vi "BuildPopupHelper.vi"(1 "new":T1(array[cluster]), 2 "main":T1(array[cluster]), 3 "Skip Count":i32) -> (0 "sum":T1(array[cluster]))   [LabVIEW 2017, in "XDataNode.xnode"]
uses:
  <vilib>/Platform/TimedLoop/XDataNode/XDataNode.xnode
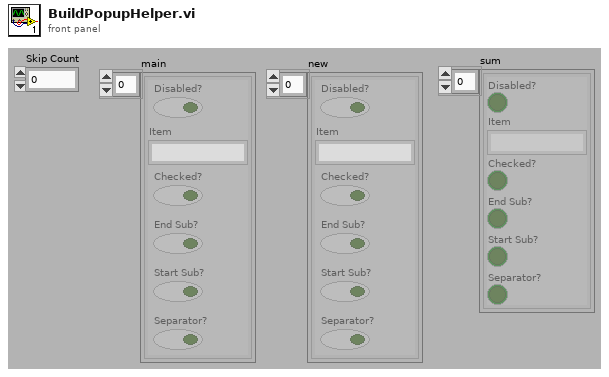
[diagram p1: front panel]
types:
  T1 = cluster{"Disabled?":bool, "Item":string, "Checked?":bool, "End Sub?":bool, "Start Sub?":bool, "Separator?":bool}[]
  T2 = cluster{"Disabled?":bool, "Item":string, "Checked?":bool, "End Sub?":bool, "Start Sub?":bool, "Separator?":bool}
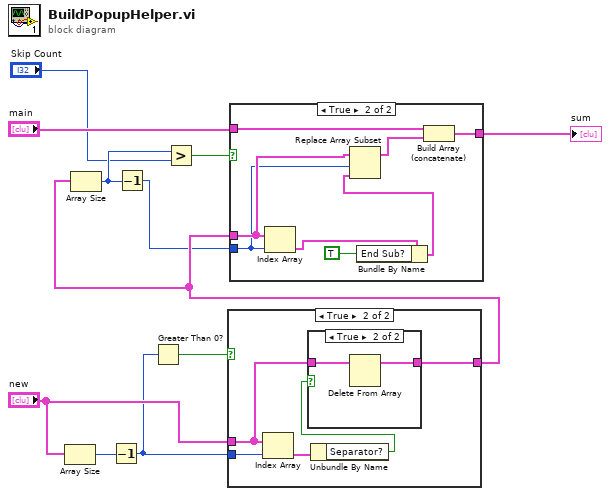
[diagram p0: block diagram]
diagram:
  n1 = Array Size(array="new") -> (size(s)=w11:i32)
  n2 = Decrement(x=w11) -> (x-1=w8:i32)
  n3 = Greater Than 0?(x=w8) -> (x > 0?=w10:bool)
  n4 = case shown="True" w10 {
    tunnel: w8 -> [_ w17]
    tunnel: "new" -> [w12 w14]
    tunnel: [w12 w13] -> w7
    frame False {
    }
    frame True {
      n5 = Index Array(array=w14, index=w17) -> (element=w16:T2)
      n6 = Unbundle By Name(w16) -> ("Separator?"=w15:bool)
      n7 = case shown="True" w15 {
        tunnel: w14 -> [w18 w20]
        tunnel: [w18 w19] -> w13
        frame False {
        }
        frame True {
          n8 = Delete From Array(array=w20) -> (array with subset deleted=w19:T1)  [unwired: 2 in, 1 out]
        }
      }
    }
  }
  n9 = Array Size(array=w7) -> (size(s)=w3:i32)
  n10 = Decrement(x=w3) -> (x-1=w6:i32)
  n11 = Greater?(x=w3, y="Skip Count") -> (0:w1:bool)
  n12 = case shown="True" w1 {
    tunnel: w6 -> [_ w27]
    tunnel: w7 -> [_ w28]
    tunnel: "main" -> [w21 w24]
    tunnel: [w21 w23] -> w4
    frame False {
    }
    frame True {
      n13 = Index Array(array=w28, index=w27) -> (element=w26:T2)
      n14 = Bundle By Name(cluster=w26, "End Sub?"=TRUE) -> (w25:T2)
      n15 = Replace Array Subset(array=w28, new element=w25, index=w27) -> (w22:T1)
      n16 = Build Array (concatenate)(w24, w22) -> (w23:T1)
    }
  }
  "sum" <- w4
